vi "Re-Init.vi"(5 "Motion Control":T8, 7 "Enum":enum16{"Circular", "Cylindrical", "Spiral"}(ring)=enum."Spiral", 8 "error in (no error)":errorcluster, 9 "# lin. steps":dbl, 10 "# rot. steps":dbl, 11 "AirSAS Controls":T1 {"Waveform"."LFM Parameters"."Window %" format="%.2g"; "Waveform"."LFM Parameters"."Out. Amplitude (Vpk)" format="%0.2f"; "Waveform"."LFM Parameters"."Fstop (Hz)" format="%^.3e"; "Waveform"."LFM Parameters"."Fstart (Hz)" format="%^.3e"; "Waveform"."LFM Parameters"."Duration" format="%.3f"}) -> (0 "error out":errorcluster, 3 "output cluster":T1={"Receive Duration"=0.0, "I/O"={"DAQmx Device"="Dev1", "AO Range"=0.0, "AI Range"=0.0, "DAQ Group Delay"=0.0, "Fs"=0.0}, "Hardware"={"Centerpos"=[0.0, 0.0, 0.0], "TXpos"=[0.0, 0.0, 0.0], "RX1pos"=[0.0, 0.0, 0.0], "RX2pos"=[0.0, 0.0, 0.0], "Angle"=0.0, "Height"=0.0}, "Waveform"={"LFM Parameters"={"Duration"=1.0, "Fstart (Hz)"=1000.0, "Fstop (Hz)"=10000.0, "Out. Amplitude (Vpk)"=1.0, "Window %"=10.0}, "Transmit Waveform"={"t0"=timestamp(0 s since 1904-01-01), "dt"=1.0, "Y"=[]}}, "LINX Resource"={"IO"=enum."Remote", "Interface"=enum."Serial", "LINX Device Config"={"Interface"=enum."Serial", "COM Port"="COM13", "TCP Configuration"={"IP Address"="", "Port"=0}, "Device Family"=1, "Device ID"=1, "Device Name"="myRIO-1900", "TCP Ref"=refnum, "Channels"={"DI"=[0, 1, 2, 3, 4, 5, 6, 7, 8, 9, 10, 11, 12, 13, 14, 15, 16, 17, 18, 19, 20, 21, 22, 23, 24, 25, 26, 27, 28, 29, 30, 31, 32, 33, 34, 35, 36, 37, 38, 39, 40, 41, 42, 43, 44, 45, 46], "DO"=[0, 1, 2, 3, 4, 5, 6, 7, 8, 9, 10, 11, 12, 13, 14, 15, 16, 17, 18, 19, 20, 21, 22, 23, 24, 25, 26, 27, 28, 29, 30, 31, 32, 33, 34, 35, 36, 37, 38, 39, 40, 41, 42, 43, 44, 45, 46], "AI"=[0, 1, 2, 3, 4, 5, 6, 7, 8, 9, 10, 11], "AO"=[], "PWM"=[3, 5, 6, 9, 10], "QE"=[], "UART"=[0, 1], "I2C 2"=[0], "SPI"=[0], "CAN"=[], "Servo"=[], "AI Ref (V)"=0.0, "AI Resolution (Bits)"=0, "AO Ref (V)"=0.0, "AO Resolution (Bits)"=0}}}, "Port"=3000.0} {"Waveform"."LFM Parameters"."Window %" format="%.2g"; "Waveform"."LFM Parameters"."Out. Amplitude (Vpk)" format="%0.2f"; "Waveform"."LFM Parameters"."Fstop (Hz)" format="%^.3e"; "Waveform"."LFM Parameters"."Fstart (Hz)" format="%^.3e"; "Waveform"."LFM Parameters"."Duration" format="%.3f"})   [LabVIEW 2018]
uses:
  N:/SRDD-Student/Ng/fromTom/Air SAS Data Acquisition/controls/Air SAS Controls.ctl
  <vilib>/MakerHub/LINX/Private/Type Defs/LINX Ref.ctl
  <vilib>/MakerHub/LINX/Private/Type Defs/Platform.ctl
  <vilib>/MakerHub/LINX/Private/Type Defs/Interface.ctl
  <vilib>/MakerHub/LINX/Private/Device/Type Defs/LINX Device Config.ctl
  <vilib>/MakerHub/LINX/Private/Device/Type Defs/TCP Config.ctl
  <vilib>/MakerHub/LINX/Private/Device/Type Defs/Channels.ctl
  <vilib>/MakerHub/LINX/LMH-LINX.lvlib
  <vilib>/MakerHub/LINX/Private/Device/Device.lvlib
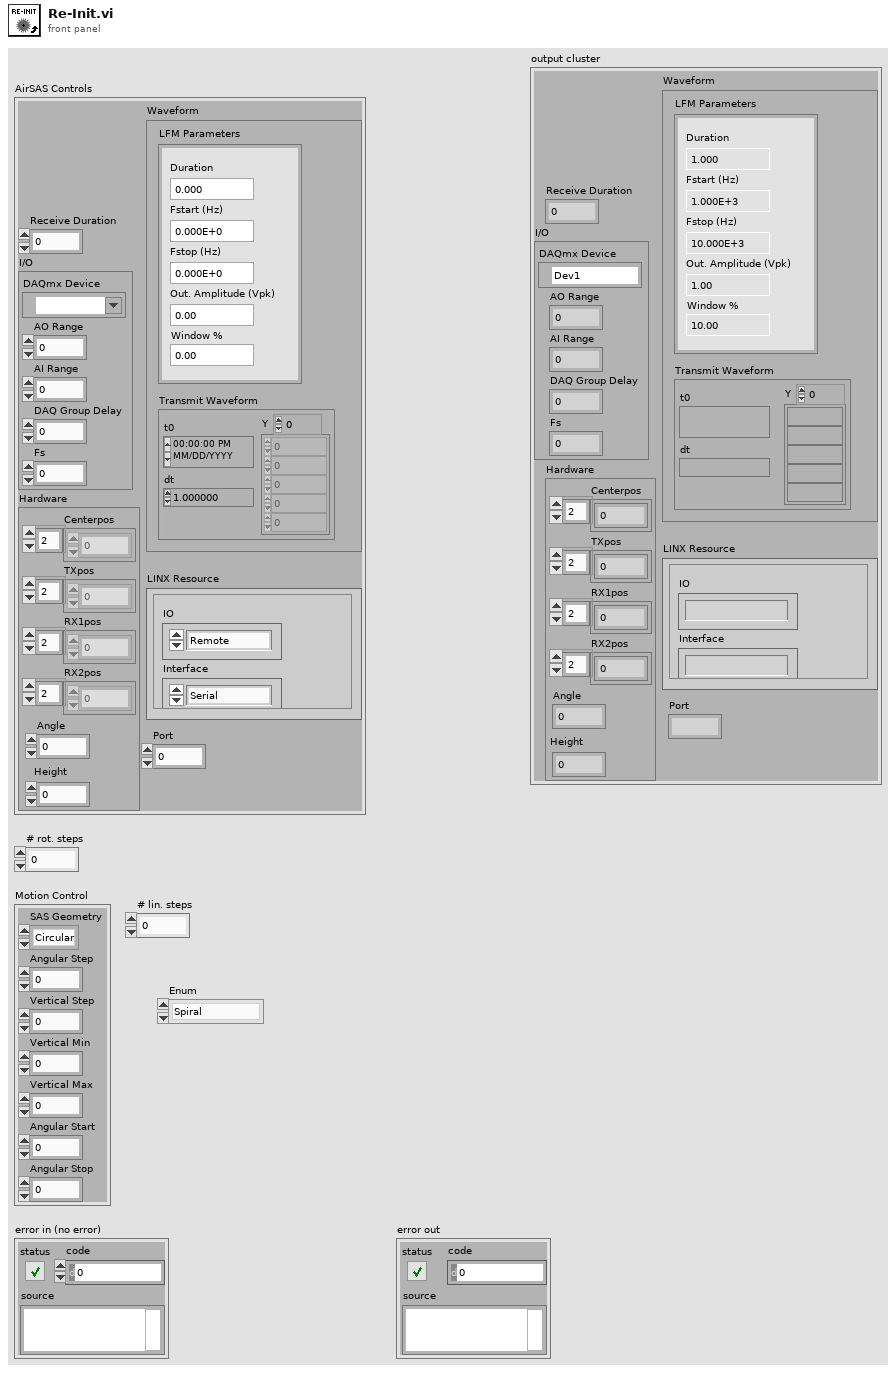
[diagram p1: front panel]
types:
  T1 = typedef "Air SAS Controls.ctl" = cluster{"Receive Duration":dbl, "I/O":cluster{"DAQmx Device":tag, "AO Range":dbl, "AI Range":dbl, "DAQ Group Delay":dbl, "Fs":dbl}, "Hardware":cluster{"Centerpos":dbl[], "TXpos":dbl[], "RX1pos":dbl[], "RX2pos":dbl[], "Angle":dbl, "Height":dbl}, "Waveform":cluster{"LFM Parameters":cluster{"Duration":dbl, "Fstart (Hz)":dbl, "Fstop (Hz)":dbl, "Out. Amplitude (Vpk)":dbl, "Window %":dbl}, "Transmit Waveform":waveform(dbl)}, "LINX Resource":T2, "Port":dbl}
  T2 = typedef "LMH-LINX.lvlib/LINX Ref.ctl" = cluster{"IO":T3, "Interface":T4, "LINX Device Config":T5}
  T3 = typedef "LMH-LINX.lvlib/Platform.ctl" = enum16{"Remote", "Local"}
  T4 = typedef "LMH-LINX.lvlib/Interface.ctl" = enum16{"Serial", "TCP"}
  T5 = typedef "LMH-LINX.lvlib/Device.lvlib/LINX Device Config.ctl" = cluster{"Interface":T4, "COM Port":refnum<visa-resource-name>, "TCP Configuration":T6, "Device Family":u8, "Device ID":u8, "Device Name":string, "TCP Ref":refnum<k5>, "Channels":T7}
  T6 = typedef "LMH-LINX.lvlib/Device.lvlib/TCP Config.ctl" = cluster{"IP Address":string, "Port":u16}
  T7 = typedef "LMH-LINX.lvlib/Channels.ctl" = cluster{"DI":u8[], "DO":u8[], "AI":u8[], "AO":u8[], "PWM":u8[], "QE":u8[], "UART":u8[], "I2C 2":u8[], "SPI":u8[], "CAN":u8[], "Servo":u8[], "AI Ref (V)":dbl, "AI Resolution (Bits)":u8, "AO Ref (V)":dbl, "AO Resolution (Bits)":u8}
  T8 = cluster{"SAS Geometry":enum16{"Circular", "Cylindrical", "Spiral"}, "Angular Step":dbl, "Vertical Step":dbl, "Vertical Min":dbl, "Vertical Max":dbl, "Angular Start":dbl, "Angular Stop":dbl}
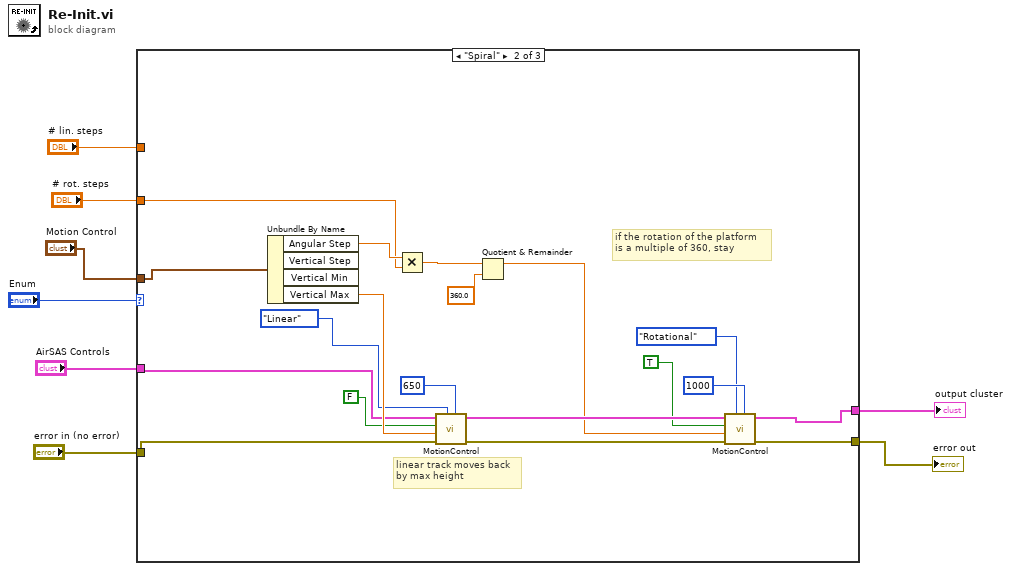
[diagram p0: block diagram]
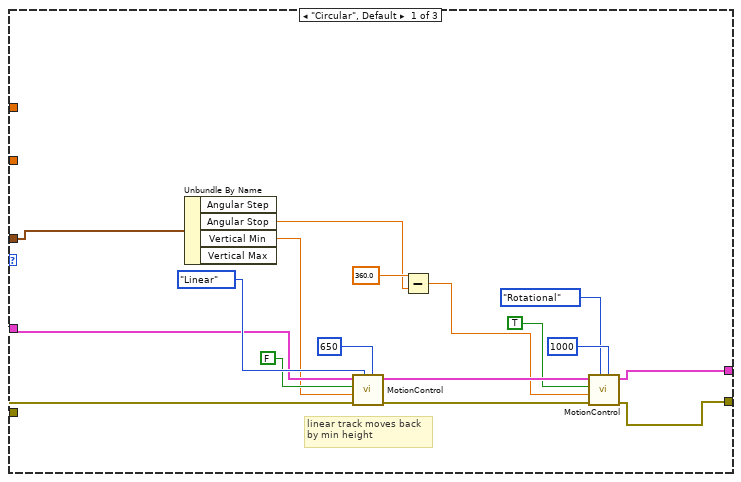
[diagram p2: hidden frame]
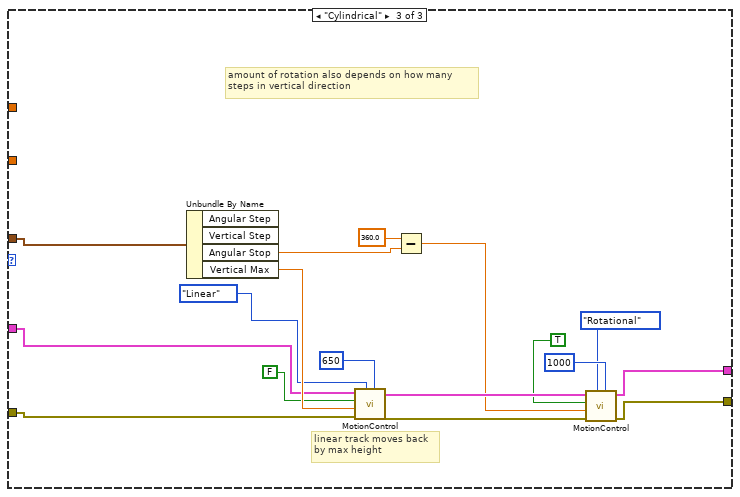
[diagram p3: hidden frame]
diagram:
  n1 = case shown="\"Spiral\"" "Enum" {
    tunnel: "# rot. steps" -> [_ w36 _]
    tunnel: "Motion Control" -> [w15 w37 w55]
    tunnel: "AirSAS Controls" -> [w20 w35 w54]
    tunnel: "error in (no error)" -> [w19 w34 w53]
    tunnel: [w17 w33 w52] -> w3
    tunnel: [w16 w32 w51] -> w2
    tunnel: "# lin. steps" -> [_ _ _]
    frame "Circular", Default {
      # "linear track moves back\nby min height"
      n2 = Unbundle By Name(w15) -> ("Angular Stop"=w10:dbl, "Vertical Min"=w18:dbl)  [unwired: 2 out]
      n3 = call "MotionControl.vi"("Frequency (Hz) 3"=u32 650, "Motion Type"=enum16{"Linear", "Rotational"}."Linear", "Error In"=w19, "Distance"=w18, "Direction"=FALSE ("Boolean"), "AirSAS Controls"=w20) -> ("Error Out"=w24:errorcluster, "output cluster"=w25:T1)  [unwired: 4 in]
      n4 = Subtract(x=360.0 ("y"), y=w10) -> (x-y=w9:dbl)
      n5 = call "MotionControl.vi"("Frequency (Hz) 3"=u32 1000, "Motion Type"=enum16{"Linear", "Rotational"}."Rotational", "Error In"=w24, "Distance"=w9, "Direction"=TRUE ("Boolean"), "AirSAS Controls"=w25) -> ("Error Out"=w16:errorcluster, "output cluster"=w17:T1)  [unwired: 4 in]
    }
    frame "Spiral" {
      # "linear track moves back\nby max height"
      # "if the rotation of the platform\nis a multiple of 360, stay"
      n6 = Unbundle By Name(w37) -> ("Angular Step"=w42:dbl, "Vertical Max"=w44:dbl)  [unwired: 2 out]
      n7 = Multiply(x=w42, y=w36) -> (x*y=w30:dbl)
      n8 = call "MotionControl.vi"("Frequency (Hz) 3"=u32 650, "Motion Type"=enum16{"Linear", "Rotational"}."Linear", "Error In"=w34, "Distance"=w44, "Direction"=FALSE ("Boolean"), "AirSAS Controls"=w35) -> ("Error Out"=w43:errorcluster, "output cluster"=w39:T1)  [unwired: 4 in]
      n9 = Quotient & Remainder(x=w30, y=360.0) -> (x-y*floor(x/y)=w26:dbl)  [unwired: 1 out]
      n10 = call "MotionControl.vi"("Frequency (Hz) 3"=u32 1000, "Motion Type"=enum16{"Linear", "Rotational"}."Rotational", "Error In"=w43, "Distance"=w26, "Direction"=TRUE ("Boolean"), "AirSAS Controls"=w39) -> ("Error Out"=w32:errorcluster, "output cluster"=w33:T1)  [unwired: 4 in]
    }
    frame "Cylindrical" {
      # "linear track moves back\nby max height"
      # "amount of rotation also depends on how many\nsteps in vertical direction"
      n11 = Unbundle By Name(w55) -> ("Angular Stop"=w49:dbl, "Vertical Max"=w61:dbl)  [unwired: 2 out]
      n12 = call "MotionControl.vi"("Frequency (Hz) 3"=u32 650, "Motion Type"=enum16{"Linear", "Rotational"}."Linear", "Error In"=w53, "Distance"=w61, "Direction"=FALSE ("Boolean"), "AirSAS Controls"=w54) -> ("Error Out"=w60:errorcluster, "output cluster"=w57:T1)  [unwired: 4 in]
      n13 = Subtract(x=360.0 ("y"), y=w49) -> (x-y=w45:dbl)
      n14 = call "MotionControl.vi"("Frequency (Hz) 3"=u32 1000, "Motion Type"=enum16{"Linear", "Rotational"}."Rotational", "Error In"=w60, "Distance"=w45, "Direction"=TRUE ("Boolean"), "AirSAS Controls"=w57) -> ("Error Out"=w51:errorcluster, "output cluster"=w52:T1)  [unwired: 4 in]
    }
  }
  "output cluster" <- w3
  "error out" <- w2
